vi "TwGetTofSpectrumFromShMem.vi"(2 "Normalize":bool, 3 "error in (no error)":errorcluster, 4 "BufIndex":i32, 5 "SegmentEndIndex":i32, 6 "SegmentIndex":i32, 7 "Tof spectrum in":sgl[](array[numeric])) -> (0 "Tof spectrum out":sgl[](array[numeric]), 1 "error out":errorcluster)   [LabVIEW 2009]
uses:
  TofDaqDll.dll
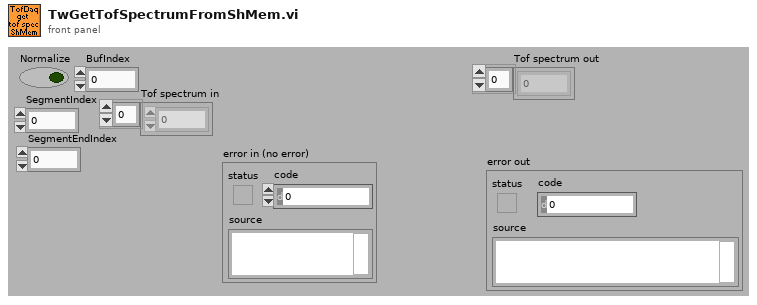
[diagram p1: front panel]
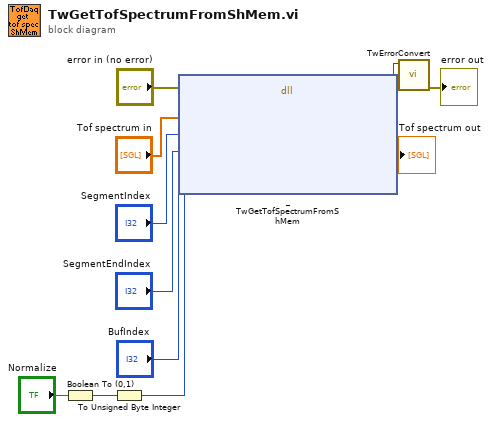
[diagram p0: block diagram]
diagram:
  n1 = Boolean To (0,1)(Boolean="Normalize") -> (0, 1=w8:i16)
  n2 = To Unsigned Byte Integer(number=w8) -> (unsigned 8bit integer=w7:u8)
  n3 = dll-call lib="C:/src/TofDaq/APIandWrappers/LabView/TofDaqDll/TofDaqDll.dll" fn="_TwGetTofSpectrumFromShMem"(error in="error in (no error)", "Spectrum"="Tof spectrum in", "SegmentIndex"="SegmentIndex", "SegmentEndIndex"="SegmentEndIndex", "BufIndex"="BufIndex", "Normalize"=w7) -> (error out=w11:errorcluster, "TwRetVal"=w10:i32, "Spectrum"=→"Tof spectrum out":sgl[])  [unwired: 6 in, 1 out]
  n4 = call "TwErrorConvert.vi"("error in (no error)"=w11, "error code"=w10) -> ("error out"=→"error out":errorcluster)  [unwired: 9 out]
